vi "pp3_DAQ_AudioLoadStimulus.vi"(0 "State Info In":T4={"Curr  tr"=0, "Curr (ms)"=0, "Cum (ms)"=0, "Run loop diff"=0, "Tone countdown (ms)"=0, "Countdown (ms)"=0, "Curr State"=enum."0 NULL", "Prev State"=enum."1 Habituation", "Rw"=FALSE, "Sw"=FALSE, "Tone\nGate"=FALSE, "Punish"=FALSE, "Current DAQ DO Int"=0, "Current Loaded Trial"={"Trial Type Number"=1, "Trial Type"=enum."GO", "Trial Weight"=100, "Shock (mA)"=0.3, "Duration (ms)"=0.25, "Sound Type"=enum."04 FM Sweep", "Stim P1"=4000.0, "Stim P2"=0.0, "Stim P3"=0.0, "Stim P4"=2000.0, "DAQ Amplitude (V)"=0.25}, "Next Trial (for display purposes)"={"Trial Type Number"=1, "Trial Type"=enum."GO", "Trial Weight"=100, "Shock (mA)"=0.3, "Duration (ms)"=0.25, "Sound Type"=enum."04 FM Sweep", "Stim P1"=4000.0, "Stim P2"=0.0, "Stim P3"=0.0, "Stim P4"=2000.0, "DAQ Amplitude (V)"=0.25}, "Total trials memo"=0, "State start cum memo (ms)"=0, "Last dur jump time memo (ms)"=0, "Last dur shock time memo (ms)"=0, "Tone repeat memo (ms)"=0, "Webcam on"=FALSE, "Webcam recording"=FALSE, "State update flag"=FALSE, "Last loaded shock voltage"=0.0, "Vid upd"=enum."0"} {"Current DAQ DO Int" format="%016b"; "Next Trial (for display purposes)"."DAQ Amplitude (V)" min=0.0 max=5.0 format="%_4g"; "Next Trial (for display purposes)"."Shock (mA)" min=-1.0 max=5.0; "Next Trial (for display purposes)"."Trial Weight" step=1; "Next Trial (for display purposes)"."Duration (ms)" min=0.0 max=1.0; "Next Trial (for display purposes)"."Trial Type Number" min=1 max=256 step=1; "Current Loaded Trial"."DAQ Amplitude (V)" min=0.0 max=5.0 format="%_4g"; "Current Loaded Trial"."Shock (mA)" min=-1.0 max=5.0; "Current Loaded Trial"."Trial Weight" step=1; "Current Loaded Trial"."Duration (ms)" min=0.0 max=1.0; "Current Loaded Trial"."Trial Type Number" min=1 max=256 step=1}, 5 "Daq config In":T1={"Sound AO"="Dev6/ao0", "Shock intesity AO"="Dev6/ao1", "Code_LED DO"="Dev6/port1:2", "Switch DI"="Dev6/port1/line0", "Webcam"="cam9", "Sound AO task"="", "Sound card task"=0, "Shock intensity AO task"="", "Code_LED DO task"="", "Switch DI task"="", "AO <=> Sound card"=FALSE, "Sound card"=0, "sample rate"=100000.0, "Variable shock"=TRUE, "Webcam on"=FALSE, "Waveform memo"={"t0"=timestamp(0 s since 1904-01-01), "dt"=1.0, "Y"=[]}, "First time"=FALSE, "Tone trigger"="", "Master-9 DO"="Dev6/port0/line5:7", "Master-9 DO task"=""} {"sample rate" min=8000.0; "Sound card task" format="%.0x"}, 11 "error in (no error)":errorcluster) -> (6 "Daq config Out":T1={"Sound AO"="Dev6/ao0", "Shock intesity AO"="Dev6/ao1", "Code_LED DO"="Dev6/port1:2", "Switch DI"="Dev6/port1/line0", "Webcam"="cam9", "Sound AO task"="", "Sound card task"=0, "Shock intensity AO task"="", "Code_LED DO task"="", "Switch DI task"="", "AO <=> Sound card"=FALSE, "Sound card"=0, "sample rate"=100000.0, "Variable shock"=TRUE, "Webcam on"=FALSE, "Waveform memo"={"t0"=timestamp(0 s since 1904-01-01), "dt"=1.0, "Y"=[]}, "First time"=FALSE, "Tone trigger"="", "Master-9 DO"="Dev6/port0/line5:7", "Master-9 DO task"=""} {"sample rate" min=8000.0; "Sound card task" format="%.0x"}, 15 "error out":errorcluster)   [LabVIEW 2013]
uses:
  <vilib>/Analysis/NI_AALBase.lvlib
  labolabo2/waveforms/WFParameters.ctl
  labolabo2/waveforms/WFRepetitions.ctl
  pp3_CTL_State.ctl
  pp3_CTL_StateInfo.ctl
  labolabo2/waveforms/WFTypes.ctl
  <vilib>/sound2/lvsound2.llb/Sound Output Task ID.ctl
  <vilib>/userdefined/High Color/IMAQdx.ctl
  pp3c_CTL_DaqStatusVariable.ctl
  pp3_CTL_TrialType.ctl
  pp3_CTL_Trial.ctl
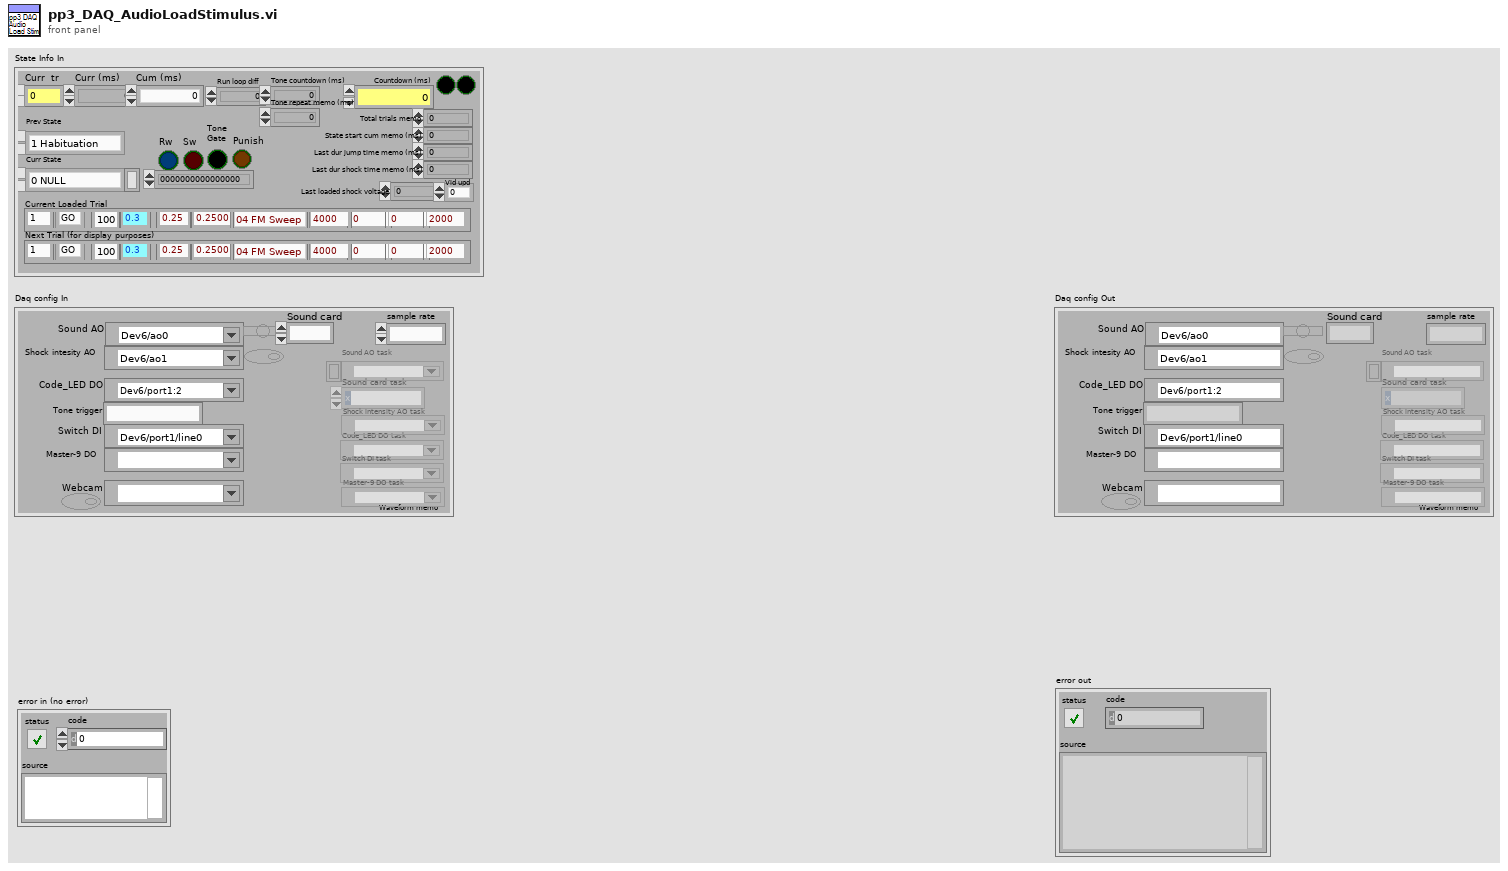
[diagram p1: front panel]
types:
  T1 = typedef "pp3c_CTL_DaqStatusVariable.ctl" = cluster{"Sound AO":tag, "Shock intesity AO":tag, "Code_LED DO":tag, "Switch DI":tag, "Webcam":T2, "Sound AO task":refnum<k21>, "Sound card task":T3, "Shock intensity AO task":refnum<k21>, "Code_LED DO task":refnum<k21>, "Switch DI task":refnum<k21>, "AO <=> Sound card":bool, "Sound card":u32, "sample rate":dbl, "Variable shock":bool, "Webcam on":bool, "Waveform memo":waveform(dbl), "First time":bool, "Tone trigger":string, "Master-9 DO":tag, "Master-9 DO task":refnum<k21>}
  T2 = typedef "IMAQdx.ctl" = refnum<k21>
  T3 = typedef "Sound Output Task ID.ctl" = u32
  T4 = typedef "pp3_CTL_StateInfo.ctl" = cluster{"Curr  tr":u16, "Curr (ms)":u32, "Cum (ms)":i64, "Run loop diff":i64, "Tone countdown (ms)":i64, "Countdown (ms)":i64, "Curr State":T5, "Prev State":T5, "Rw":bool, "Sw":bool, "Tone\nGate":bool, "Punish":bool, "Current DAQ DO Int":u16, "Current Loaded Trial":T6, "Next Trial (for display purposes)":T6, "Total trials memo":i64, "State start cum memo (ms)":i64, "Last dur jump time memo (ms)":i64, "Last dur shock time memo (ms)":i64, "Tone repeat memo (ms)":i64, "Webcam on":bool, "Webcam recording":bool, "State update flag":bool, "Last loaded shock voltage":dbl, "Vid upd":enum16{"0", "1", "2", "3", "4", "5", "6", "7", "8", "9"}}
  T5 = typedef "pp3_CTL_State.ctl" = enum8{"0 NULL", "1 Habituation", "2 (Load Trial)", "3 Stay Period", "4 Load Audio/Click Delay", "5 GO Trial", "6 GO Jumped", "7 GO Timeout", "8 NOGO Trial", "9 NOGO Jumped", "10 NOGO Timeout", "11 TEST Trial", "12 TEST Jumped", "13 TEST Timeout", "14 Intertrial Interval", "15 Done"}
  T6 = typedef "pp3_CTL_Trial.ctl" = cluster{"Trial Type Number":i16, "Trial Type":T7, "Trial Weight":u32, "Shock (mA)":dbl, "Duration (ms)":dbl, "Sound Type":T8, "Stim P1":dbl, "Stim P2":dbl, "Stim P3":dbl, "Stim P4":dbl, "DAQ Amplitude (V)":dbl}
  T7 = typedef "pp3_CTL_TrialType.ctl" = enum16{"OFF", "GO", "NOGO", "TEST"}
  T8 = typedef "WFTypes.ctl" = enum16{"00 NULL", "01 DC", "02 Noise", "03 Pure Tone", "04 FM Sweep"}
  T9 = typedef "WFParameters.ctl" = cluster{"Fs (Hz)":dbl, "Amp (V)":dbl, "Ramp (s)":dbl, "Dur (s)":dbl}
  T10 = typedef "WFRepetitions.ctl" = cluster{"Del (s)":dbl, "Int (s)":dbl, "N":i32}
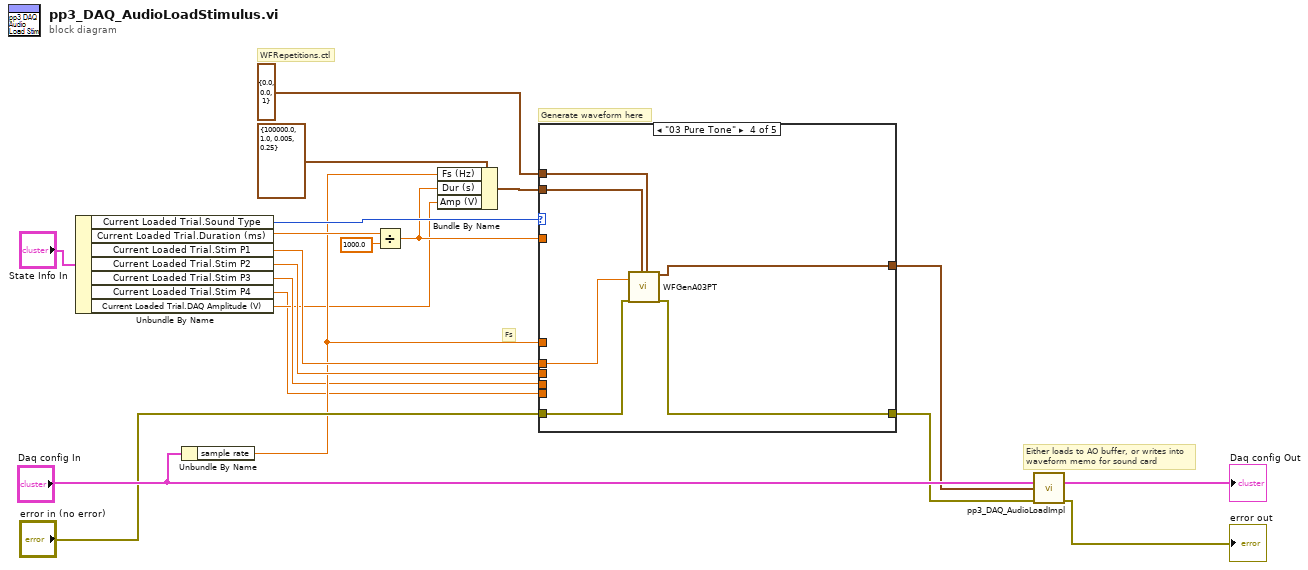
[diagram p0: block diagram]
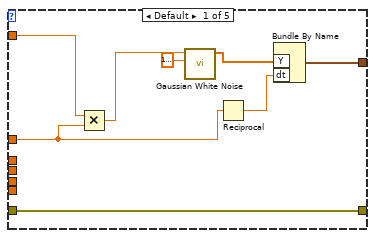
[diagram p2: hidden frame]
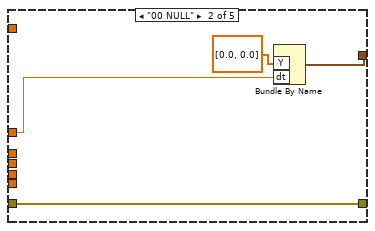
[diagram p3: hidden frame]
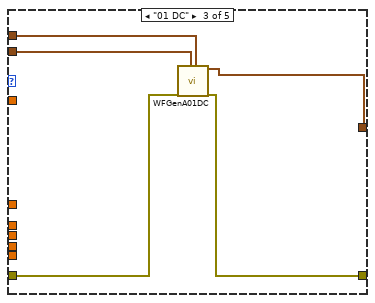
[diagram p4: hidden frame]
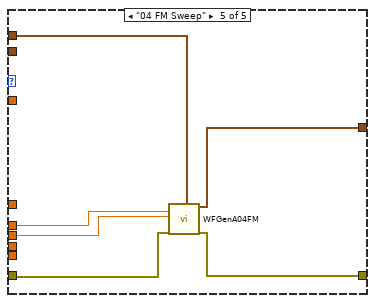
[diagram p5: hidden frame]
diagram:
  # "Fs"
  # "WFRepetitions.ctl"
  # "Either loads to AO buffer, or writes into\nwaveform memo for sound card"
  # "Generate waveform here"
  n1 = Unbundle By Name("State Info In") -> ("Current Loaded Trial.Sound Type"=w19:T8, "Current Loaded Trial.Duration (ms)"=w10:dbl, "Current Loaded Trial.Stim P1"=w12:dbl, "Current Loaded Trial.Stim P2"=w11:dbl, "Current Loaded Trial.Stim P3"=w4:dbl, "Current Loaded Trial.Stim P4"=w1:dbl, "Current Loaded Trial.DAQ Amplitude (V)"=w2:dbl)
  n2 = Unbundle By Name("Daq config In") -> ("sample rate"=w5:dbl)
  n3 = Divide(x=w10, y=1000.0) -> (x/y=w3:dbl)
  n4 = Bundle By Name(cluster=T9 {"Fs (Hz)"=100000.0, "Amp (V)"=1.0, "Ramp (s)"=0.005, "Dur (s)"=0.25} ("WFParameters"), "Fs (Hz)"=w5, "Dur (s)"=w3, "Amp (V)"=w2) -> (w7:T9)
  n5 = case shown="\"03 Pure Tone\"" w19 {
    tunnel: w5 -> [w24 w30 _ _ _]
    tunnel: [w23 w31 w35 w39 w46] -> w14
    tunnel: "error in (no error)" -> [w22 w32 w33 w41 w47]
    tunnel: [w22 w32 w34 w40 w45] -> w16
    tunnel: w12 -> [_ _ _ w38 w49]
    tunnel: w11 -> [_ _ _ _ w48]
    tunnel: T10 {"Del (s)"=0.0, "Int (s)"=0.0, "N"=1} ("WFRepetitions") -> [_ _ w36 w42 w44]
    tunnel: w7 -> [_ _ w37 w43 _]
    tunnel: w4 -> [_ _ _ _ _]
    tunnel: w3 -> [w21 _ _ _ _]
    tunnel: w1 -> [_ _ _ _ _]
    frame Default {
      n6 = Multiply(x=w21, y=w24) -> (x*y=w27:dbl)
      n7 = call <vilib>:"Gaussian White Noise.vi"("standard deviation"=1.0000000000000002, "samples"=w27) -> ("Gaussian noise pattern"=w26:dbl[])  [unwired: 8 in, 1 out]
      n8 = Reciprocal(x=w24) -> (1/x=w25:dbl)
      n9 = Bundle By Name("Y"=w26, "dt"=w25) -> (w23:waveform(dbl))  [unwired: 1 in]
    }
    frame "00 NULL" {
      n10 = Bundle By Name("Y"=dbl[] [0.0, 0.0], "dt"=w30) -> (w31:waveform(dbl))  [unwired: 1 in]
    }
    frame "01 DC" {
      n11 = call "WFGenA01DC.vi"("error in (no error)"=w33, "WFParameters"=w37, "WFRepetitions"=w36) -> ("Waveform Out"=w35:waveform(dbl), "error out"=w34:errorcluster)  [unwired: 15 in]
    }
    frame "03 Pure Tone" {
      n12 = call "WFGenA03PT.vi"("Param 0: Frequency"=w38, "error in (no error)"=w41, "WFParameters"=w43, "WFRepetitions"=w42) -> ("Waveform Out"=w39:waveform(dbl), "error out"=w40:errorcluster)  [unwired: 14 in]
    }
    frame "04 FM Sweep" {
      n13 = call "WFGenA04FM.vi"("Param 0: Start Hz"=w49, "Param 1: End Hz"=w48, "error in (no error)"=w47, "WFRepetitions"=w44) -> ("Waveform Out"=w46:waveform(dbl), "error out"=w45:errorcluster)  [unwired: 14 in]
    }
  }
  n14 = call "pp3_DAQ_AudioLoadImpl.vi"("Daq config In"="Daq config In", "Waveform"=w14, "error in (no error)"=w16) -> ("Daq config Out"=→"Daq config Out":T1, "error out"=→"error out":errorcluster)  [unwired: 11 in]
